vi "util_FilterLookup.vi"(0 "Serial Port":i32, 2 "Position (Simulate)":i32) -> (7 "Transmission":dbl)   [LabVIEW 2012]
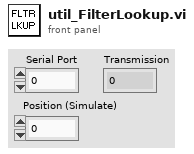
[diagram p1: front panel]
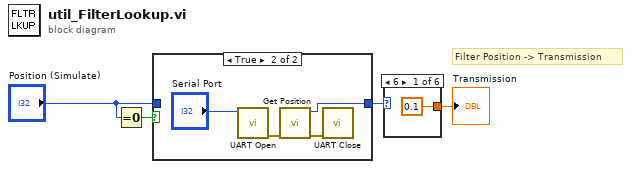
[diagram p0: block diagram]
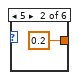
[diagram p3: hidden frame]
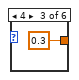
[diagram p4: hidden frame]
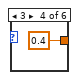
[diagram p5: hidden frame]
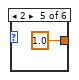
[diagram p6: hidden frame]
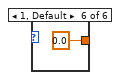
[diagram p7: hidden frame]
diagram:
  # "Filter Position -> Transmission"
  n1 = Equal To 0?(x="Position (Simulate)") -> (x = 0?=w3:bool)
  n2 = case shown="True" w3 {
    tunnel: [w5 w6] -> w2
    tunnel: "Position (Simulate)" -> [w5 _]
    frame False {
    }
    frame True {
      n3 = call "UART Open.vi"("Serial Port"="Serial Port") -> ("error out"=w9:errorcluster)  [unwired: 9 in, 1 out]
      n4 = call "Get Position.vi"("error in (no error)"=w9) -> ("error out"=w8:errorcluster, "Position"=w6:i32)  [unwired: 9 in]
      n5 = call "UART Close.vi"("error in (no error)"=w8) -> ()  [unwired: 10 in, 1 out]
    }
  }
  n6 = case shown="6" w2 {
    tunnel: [0.1 0.2 0.3 0.4 1.0 0.0] -> w4
    frame 6 {
    }
    frame 5 {
    }
    frame 4 {
    }
    frame 3 {
    }
    frame 2 {
    }
    frame 1, Default {
    }
  }
  "Transmission" <- w4
